vi "Example - Basic IPS-MC.vi"(0 "Mag_Ref":T2, 1 "MB1.T1_Ref":T2, 2 "Temp_present?":bool, 3 "LVL_present?":bool, 4 "Action":T6(ring), 5 "error in (no error)":errorcluster, 6 "LVL_Ref":T2, 7 "ISOBUS address":T5=-1, 8 "Ramp Controls":T9 {"Target Rate (T/min)" format="%_5g"; "Target Field (T)" format="%_5g"; "Target Rate (A/min)" format="%_5g"; "Target Current (A)" format="%_5g"}, 9 "Interval between messages (ms)":i16=100, 10 "Magnet Controls":T10, 11 "Range data":T1, 12 "Display Units":bool caption="AMP/TESLA", 13 "SWITCH\nHEATER":bool) -> (14 "Mag_data":T8 {"Output Voltage (V)" format="%.4f"; "Magnet Current (A)" format="%.4g"; "Output Current (A)" format="%.4g"}, 15 "Environment_data":T7 {"Nitrogen Level (%)" format="%_4f"; "Helium Level (%)" format="%_4f"; "Temperature (K)" format="%_4f"}, 16 "Status":string, 17 "Mode":string, 18 "SW HTR\nCONFIRM":bool, 19 "error out":errorcluster)   [LabVIEW 2013, in "Mercury iXX.lvlib"]
uses:
  Mercury iXX.lvlib
  Public/Libraries/Magnet/Signals/Read/Switch Heater Status (Read).vi
  Public/Libraries/Magnet.lvlib
  Public/Libraries/Magnet/Signals/Read/Current (Read).vi
  Public/Libraries/Magnet/Signals/Read/Persistant Current (Read).vi
  Public/Libraries/Temperature/Signals/Read/Temperature (Read).vi
  Public/Libraries/Temperature.lvlib
  Public/Libraries/Magnet/Configuration/Read/PSU Action Status (Read).vi
  Public/Libraries/Level Meter/Signals/Read/Probe Level Helium (Read).vi
  Public/Libraries/Level Meter.lvlib
  Public/Libraries/Level Meter/Signals/Read/Probe Level Nitrogen (Read).vi
  Public/Libraries/Magnet/Configuration/Read/PSU Status (Read).vi
  Public/Libraries/System/Read/DateTime (Read).vi
  Public/Libraries/System.lvlib
  Public/Libraries/Magnet/Signals/Read/Voltage (Read).vi
  Public/Libraries/Magnet/Controls/PSU Actions.ctl
  Public/Libraries/Magnet/Configuration/Set/PSU Action Status (Set).vi
  Public/Libraries/Magnet/Controls/Switch Heater.ctl
  Public/Libraries/Magnet/Signals/Set/Switch Heater No Check (Set).vi
  Public/Libraries/Magnet/Signals/Set/Target Current (Set).vi
  Public/Libraries/Magnet/Signals/Set/Target Current Rate (Set).vi
  Public/Libraries/Magnet/Signals/Set/Target Field (Set).vi
  Public/Libraries/Magnet/Signals/Set/Target Field Rate (Set).vi
  Public/Controls/Comms Transport Layer.ctl
  Private/Controls/Query Dynamic Reference.ctl
  Public/Controls/Mercury Reference.ctl
  Public/Controls/ISOBus Address.ctl
panel:
  out "Switch TS":timestamp
  out "System Time":string
  in  "Tab Control":enum32{"Link Panel", "Front_Panel", "Error"}(tab)
  out "Voltage (V)":dbl(knob) scale=-10.0..10.0
  out "Current (A)":dbl(knob) scale=-60.0..60.0
  in  "Sw Delay (s)":dbl=30.0 caption="Time Target (s)"
  out "Elapsed\nTime (s)":dbl caption="Elapsed Time (s)"
  out "Magnet Centre Field (T)":dbl format="%.4f"
  out "Output (T) (Field equivalent)":dbl format="%.4f"
  # "Switch Controls"
  # "MercuryiPS-VI"
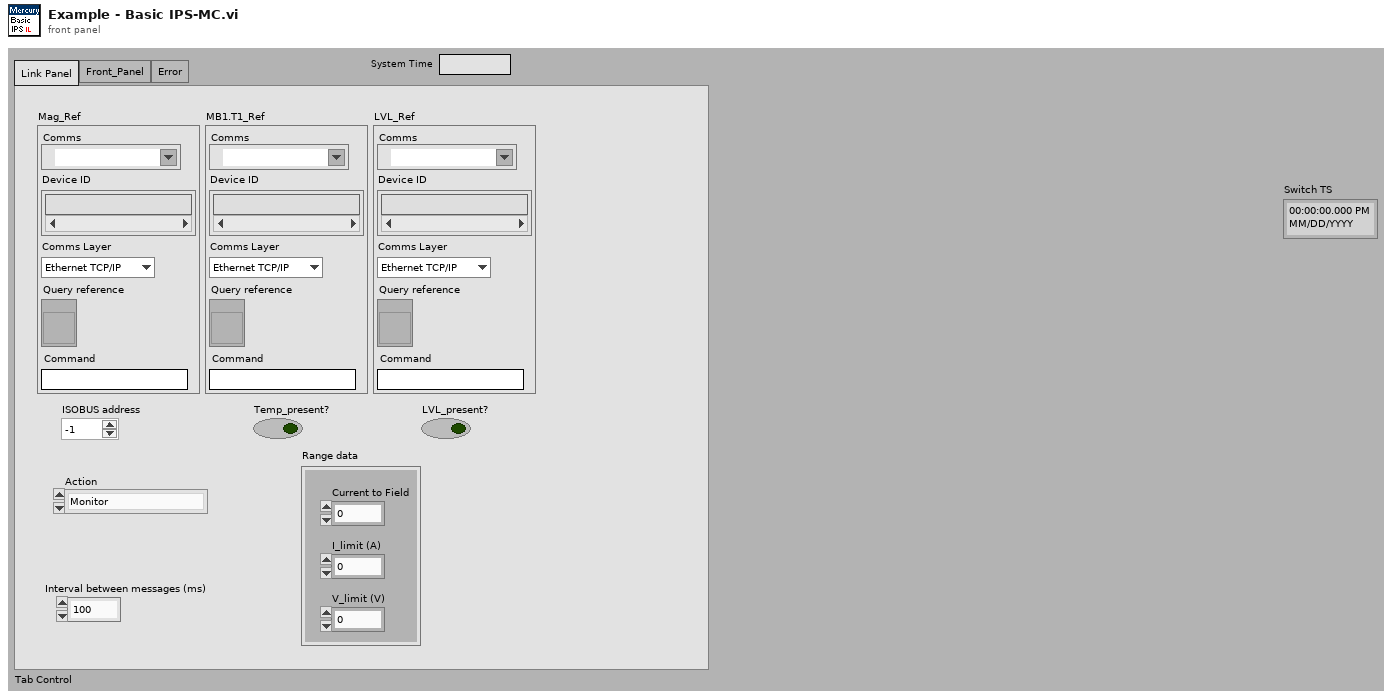
[diagram p1: front panel]
types:
  T1 = cluster{"I_limit (A)":dbl, "V_limit (V)":dbl, "Current to Field":dbl}
  T2 = typedef "Mercury iXX.lvlib/Mercury Reference.ctl" = cluster{"Comms":refnum<visa-resource-name>, "Device ID":string[], "Comms Layer":T3, "Command":string, "Query reference":T4}
  T3 = typedef "Mercury iXX.lvlib/Comms Transport Layer.ctl" = enum16{"Ethernet TCP/IP", "USB", "ISOBus - RS-232", "GPIB"}
  T4 = typedef "Mercury iXX.lvlib/Query Dynamic Reference.ctl" = refnum<vi>
  T5 = typedef "Mercury iXX.lvlib/ISOBus Address.ctl" = i32
  T6 = enum16{"Monitor", "Hold", "Clamp", "To Set", "To Zero", "Switch Heater", "Set Points"}
  T7 = cluster{"Temperature (K)":dbl, "Helium Level (%)":dbl, "Nitrogen Level (%)":dbl}
  T8 = cluster{"Output Current (A)":dbl, "Magnet Current (A)":dbl, "Output Voltage (V)":dbl}
  T9 = cluster{"Target Current (A)":dbl, "Target Rate (A/min)":dbl, "Target Field (T)":dbl, "Target Rate (T/min)":dbl}
  T10 = cluster{"CLAMP":bool, "HOLD":bool, "TO SET":bool, "TO ZERO":bool}
  T11 = typedef "Mercury iXX.lvlib/Magnet.lvlib/PSU Actions.ctl" = string
  T12 = typedef "Mercury iXX.lvlib/Magnet.lvlib/Switch Heater.ctl" = string
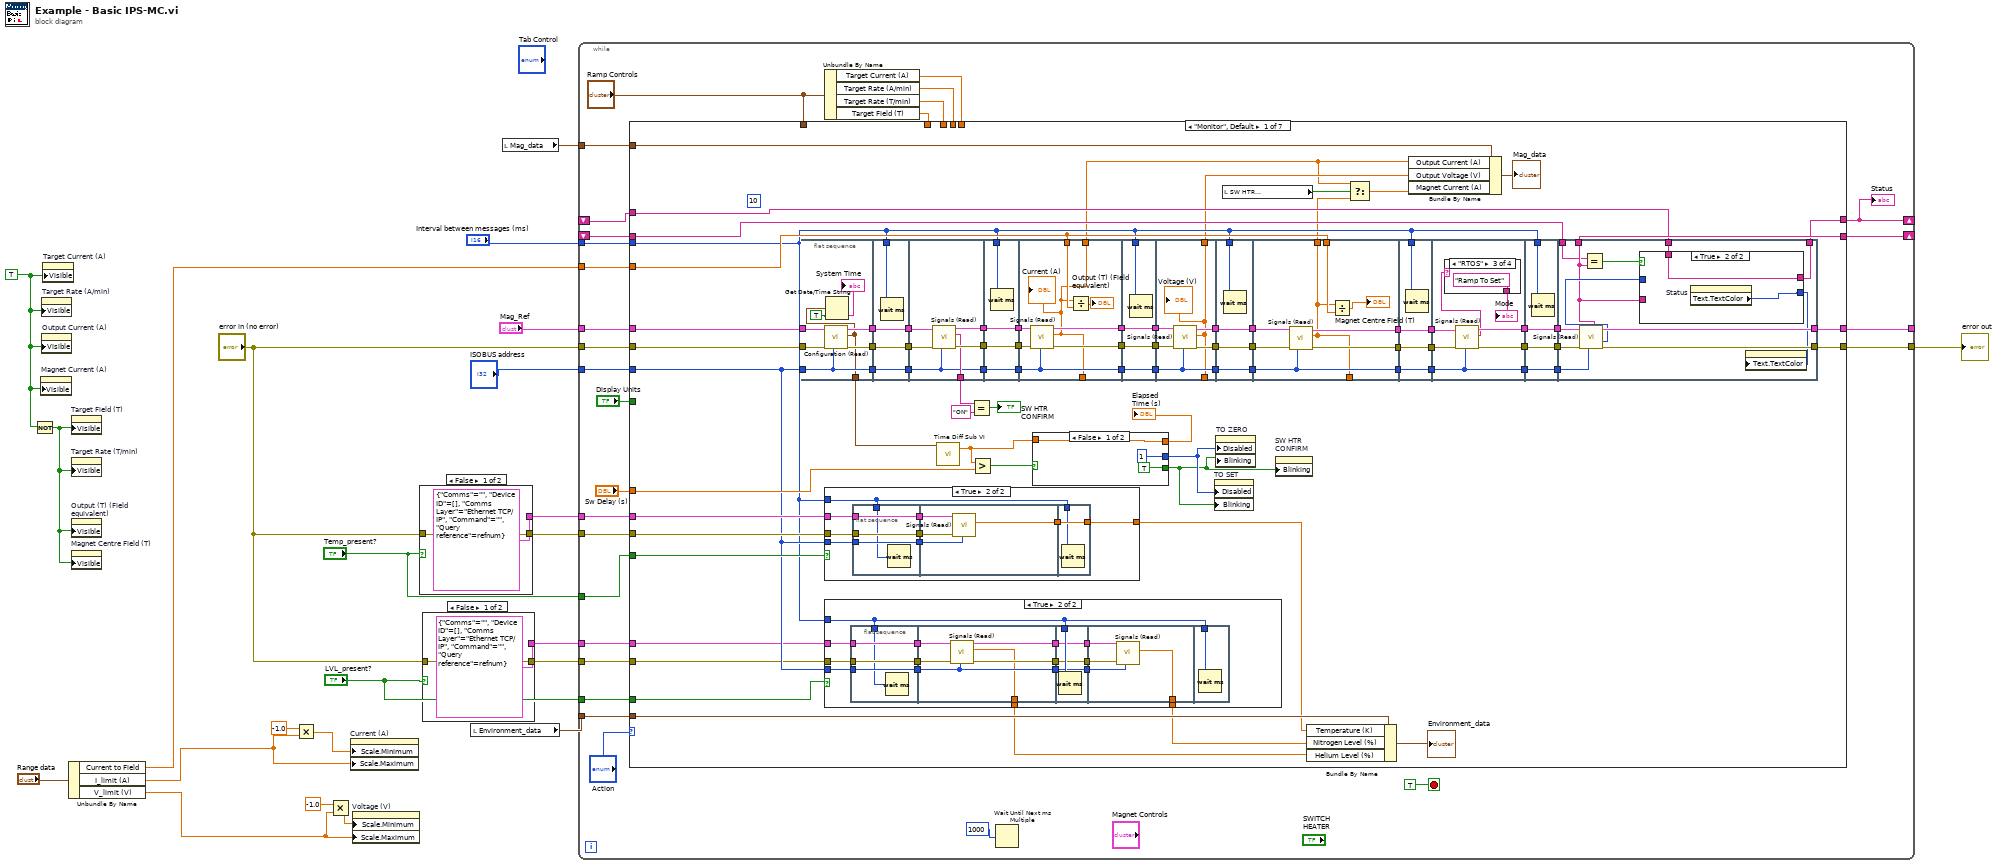
[diagram p0: block diagram]
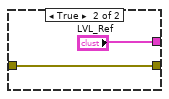
[diagram p2: hidden frame]
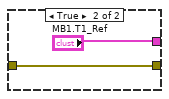
[diagram p3: hidden frame]
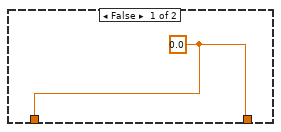
[diagram p4: hidden frame]
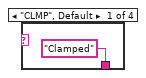
[diagram p5: hidden frame]
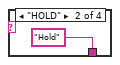
[diagram p6: hidden frame]
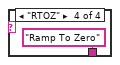
[diagram p7: hidden frame]
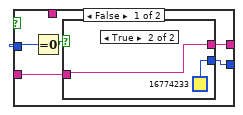
[diagram p8: hidden frame]
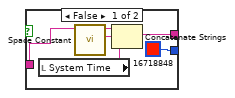
[diagram p9: hidden frame]
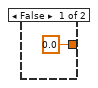
[diagram p10: hidden frame]
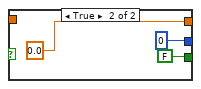
[diagram p11: hidden frame]
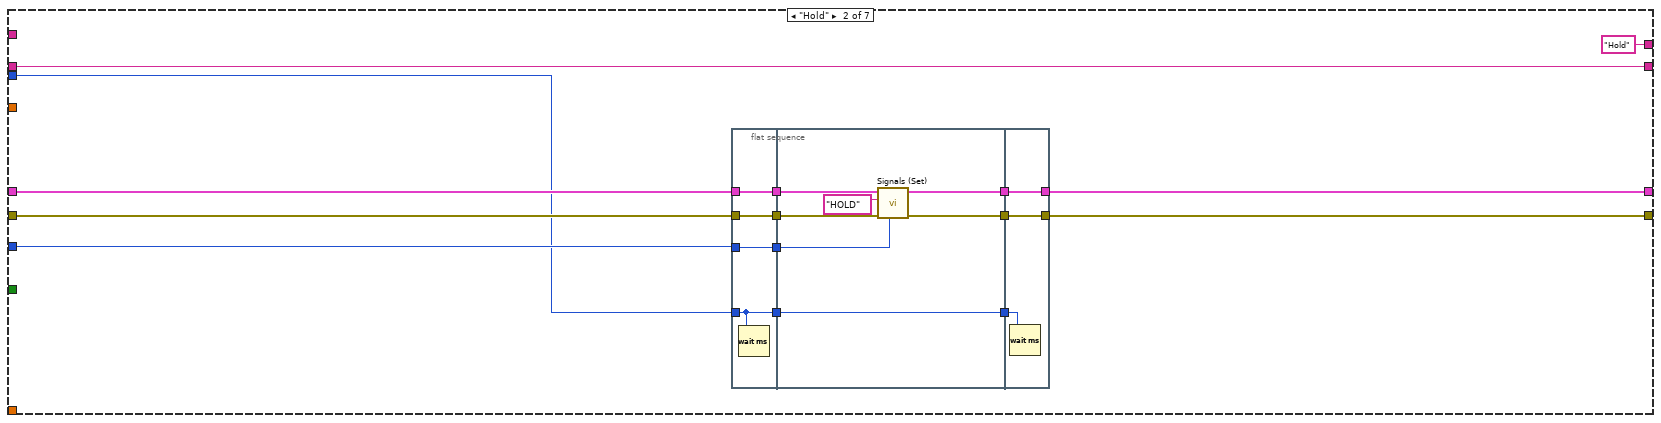
[diagram p12: hidden frame]
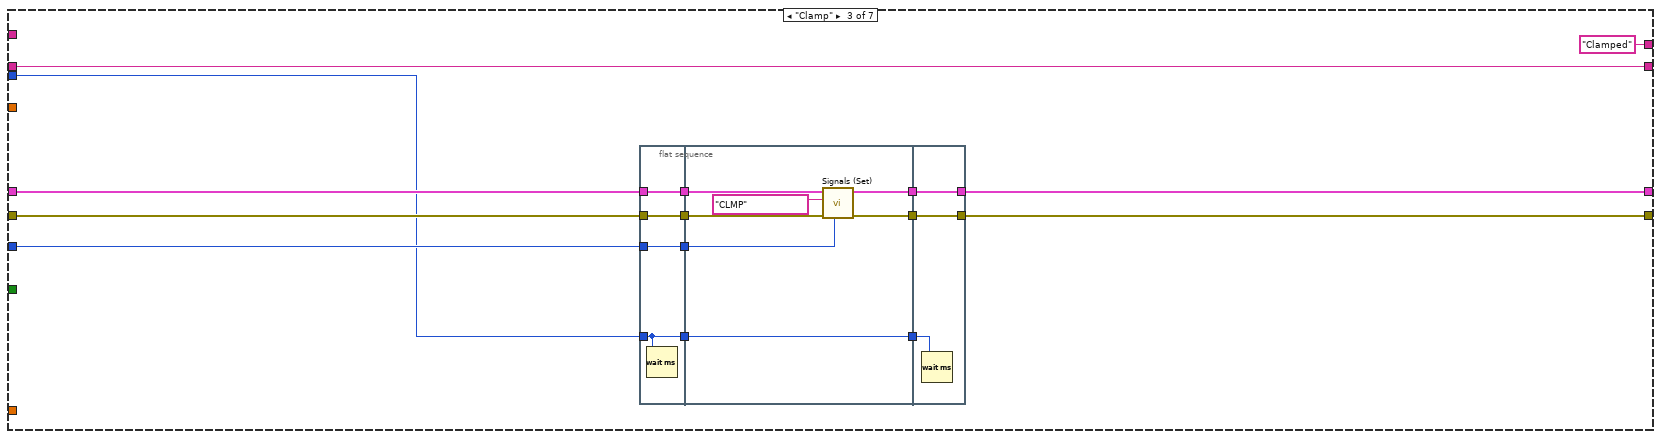
[diagram p13: hidden frame]
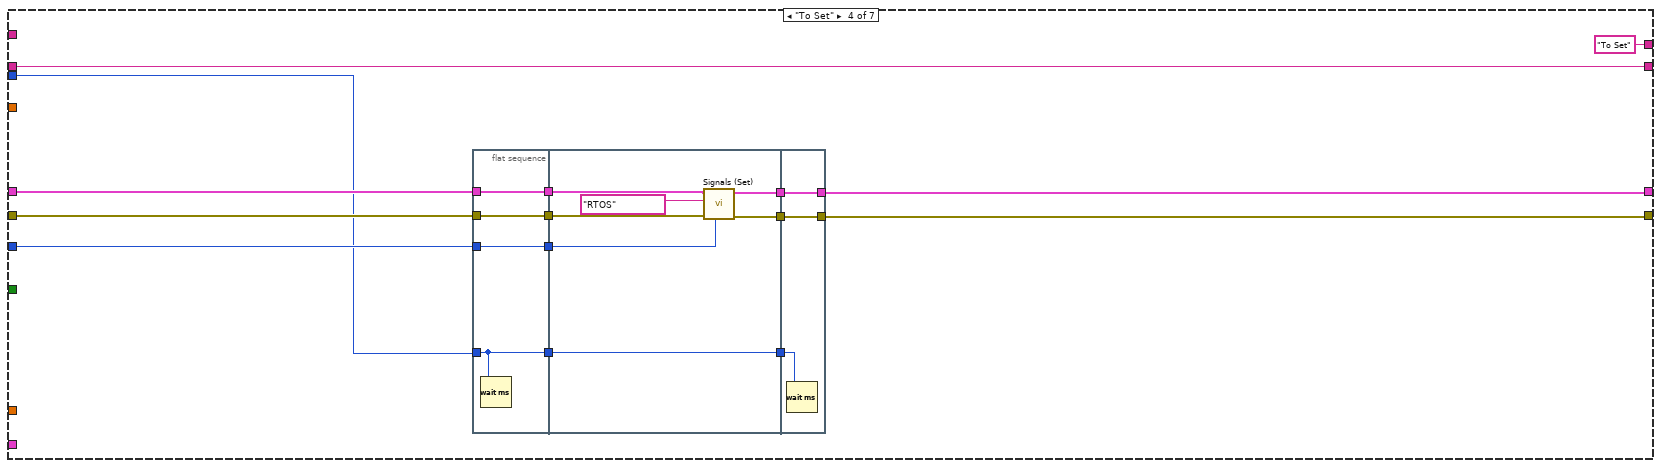
[diagram p14: hidden frame]
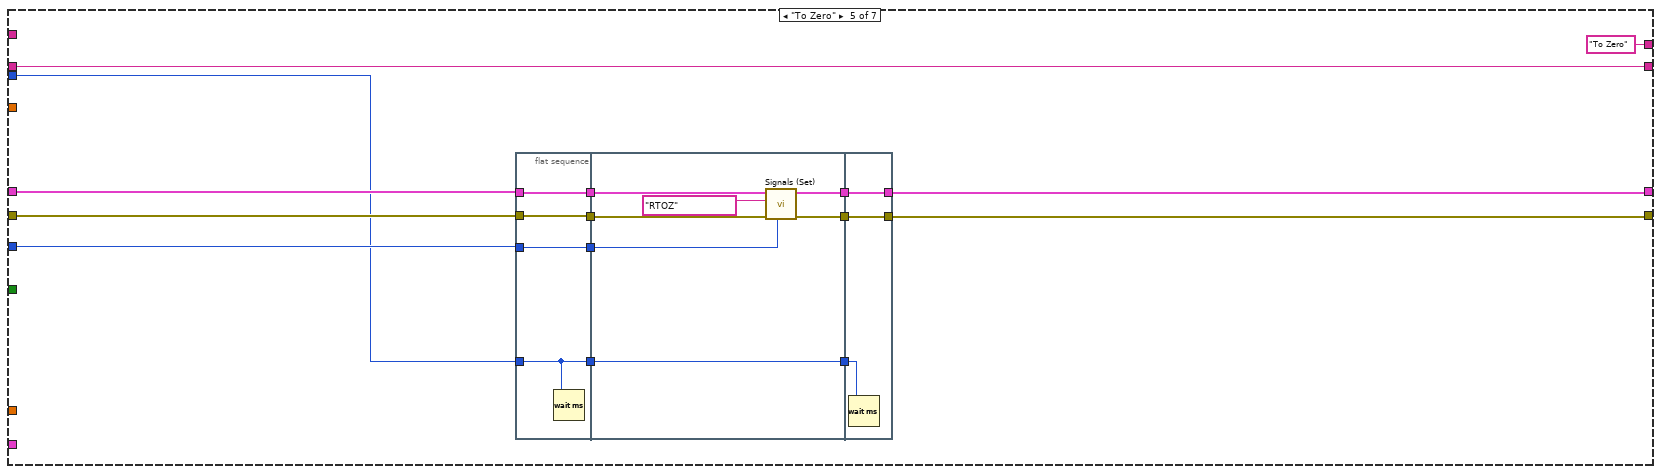
[diagram p15: hidden frame]
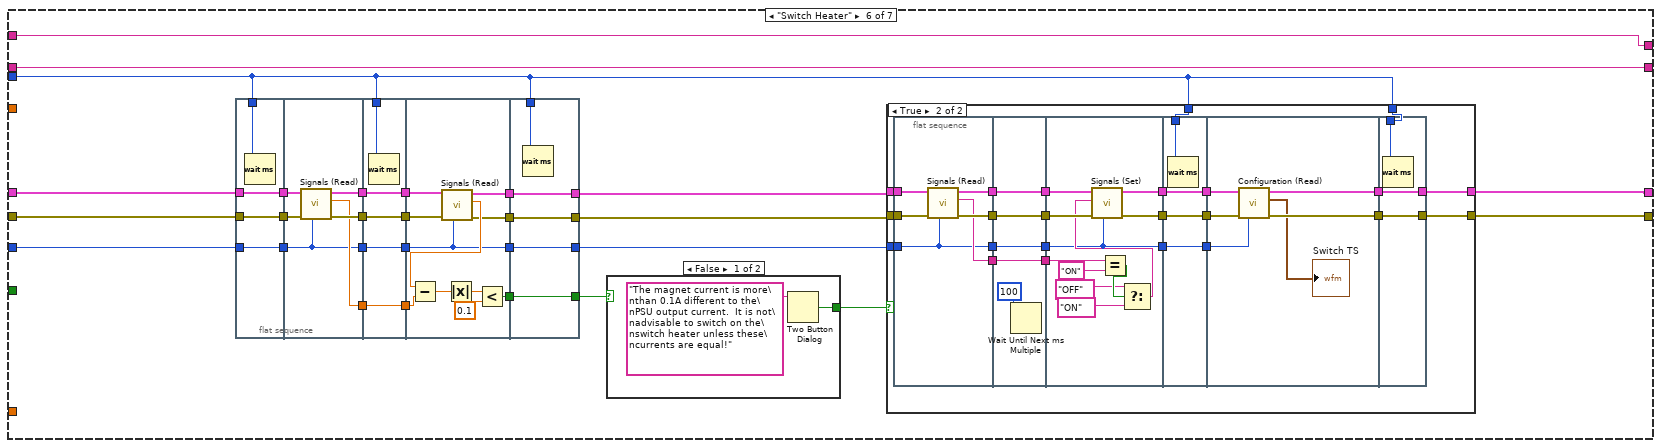
[diagram p16: hidden frame]
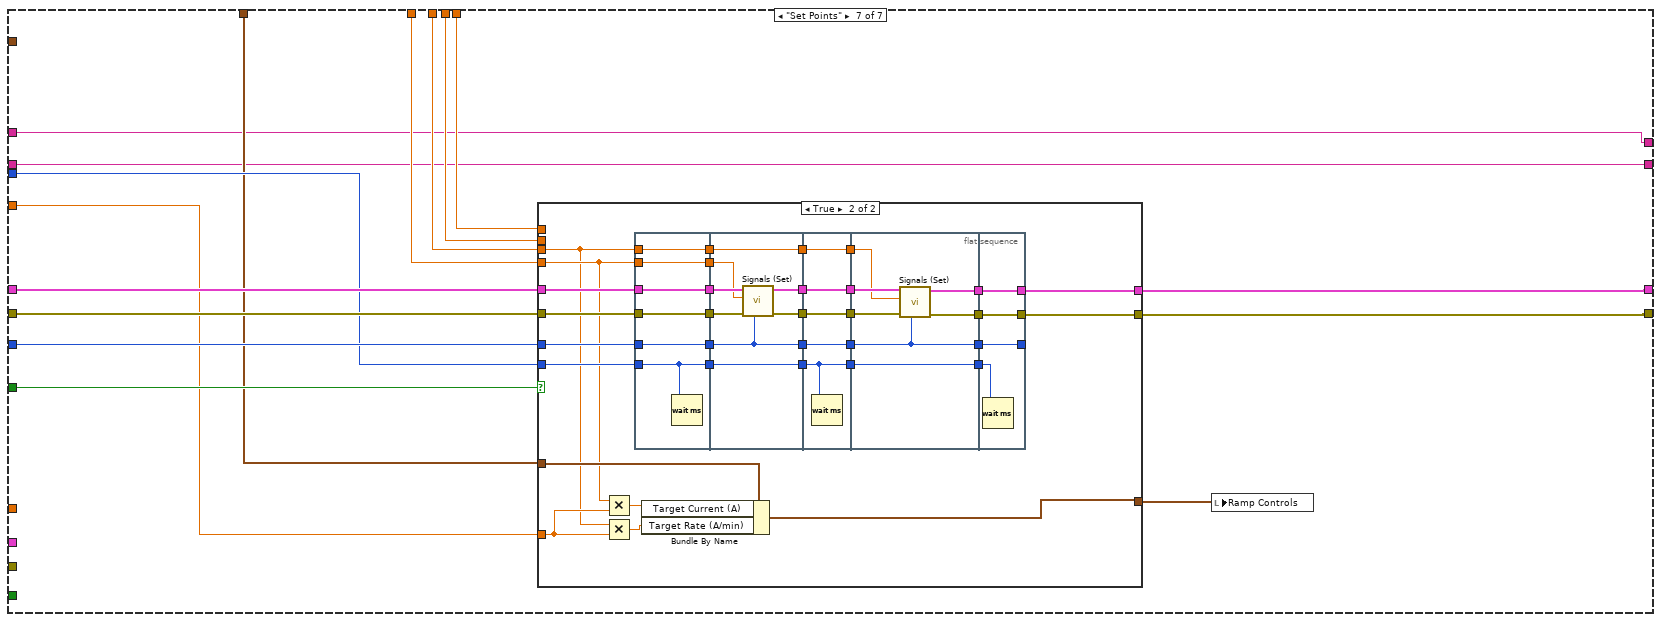
[diagram p19: hidden frame]
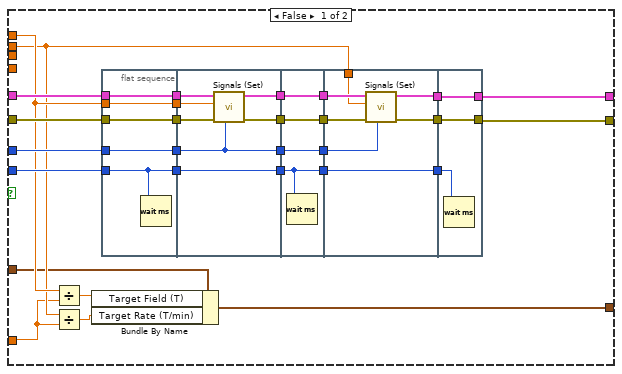
[diagram p20: hidden frame]
diagram:
  w23 = TRUE ("Visible")
  n1 = Not(x=w23) -> (.not. x?=w22:bool)
  n2 = property on="Magnet Current (A)" class="DigNum (strict)"("Visible"=w23) -> ()  [unwired: 2 in, 2 out]
  n3 = property on="Target Rate (A/min)" class="DigNum (strict)"("Visible"=w23) -> ()  [unwired: 2 in, 2 out]
  n4 = property on="Output Current (A)" class="DigNum (strict)"("Visible"=w23) -> ()  [unwired: 2 in, 2 out]
  n5 = property on="Target Current (A)" class="DigNum (strict)"("Visible"=w23) -> ()  [unwired: 2 in, 2 out]
  n6 = Unbundle By Name("Range data") -> ("Current to Field"=w2:dbl, "I_limit (A)"=w4:dbl, "V_limit (V)"=w3:dbl)
  n7 = property on="Target Field (T)" class="DigNum (strict)"("Visible"=w22) -> ()  [unwired: 2 in, 2 out]
  n8 = property on="Target Rate (T/min)" class="DigNum (strict)"("Visible"=w22) -> ()  [unwired: 2 in, 2 out]
  n9 = property on="Output (T) (Field equivalent)" class="DigNum (strict)"("Visible"=w22) -> ()  [unwired: 2 in, 2 out]
  n10 = property on="Magnet Centre Field (T)" class="DigNum (strict)"("Visible"=w22) -> ()  [unwired: 2 in, 2 out]
  n11 = Multiply(x=-1.0, y=w4) -> (x*y=w9:dbl)
  n12 = Multiply(x=-1.0, y=w3) -> (x*y=w10:dbl)
  n13 = property on="Current (A)" class="Knob (strict)"("Scale.Minimum"=w9, "Scale.Maximum"=w4) -> ()  [unwired: 2 in, 2 out]
  n14 = property on="Voltage (V)" class="Knob (strict)"("Scale.Minimum"=w10, "Scale.Maximum"=w3) -> ()  [unwired: 2 in, 2 out]
  n15 = case shown="False" "Temp_present?" {
    tunnel: "error in (no error)" -> [w25 w26]
    tunnel: [T2 {"Comms"="", "Device ID"=[], "Comms Layer"=enum."Ethernet TCP/IP", "Command"="", "Query reference"=refnum} ("MB1.T1_Ref") "MB1.T1_Ref"] -> w14
    tunnel: [w25 w26] -> w20
    frame False {
    }
    frame True {
    }
  }
  n16 = case shown="False" "LVL_present?" {
    tunnel: "error in (no error)" -> [w29 w30]
    tunnel: [T2 {"Comms"="", "Device ID"=[], "Comms Layer"=enum."Ethernet TCP/IP", "Command"="", "Query reference"=refnum} ("LVL_Ref") "LVL_Ref"] -> w19
    tunnel: [w29 w30] -> w18
    frame False {
    }
    frame True {
    }
  }
  n17 = local read "Environment_data"() -> (w16:T7)
  n18 = local read "Mag_data"() -> (w17:T8)
  n19 = while {
    tunnel: "Mag_Ref" -> [w59]
    tunnel: "error in (no error)" -> [w58]
    tunnel: [w57] -> _
    tunnel: [w56] -> w1
    tunnel: w2 -> [w54]
    tunnel: w14 -> [w47]
    tunnel: w20 -> [w46]
    tunnel: "Temp_present?" -> [w48]
    tunnel: "ISOBUS address" -> [w45]
    tunnel: "Interval between messages (ms)" -> [w44]
    tunnel: w19 -> [w43]
    tunnel: w18 -> [w42]
    tunnel: "LVL_present?" -> [w41]
    shift-right: [w40] -> _
    shift-left: _ -> [w39]
    shift-right: [w35] -> _
    shift-left: _ -> [w38]
    tunnel: w17 -> [w33]
    tunnel: w16 -> [w32]
    stop <- TRUE stop-if-true
    n20 = Unbundle By Name("Ramp Controls") -> ("Target Current (A)"=w51:dbl, "Target Rate (A/min)"=w52:dbl, "Target Rate (T/min)"=w50:dbl, "Target Field (T)"=w49:dbl)
    n21 = case shown="\"Monitor\", Default" "Action" {
      tunnel: w59 -> [w135 w301 w330 w359 w388 w422 w547]
      tunnel: w58 -> [w134 w300 w329 w358 w387 w421 w546]
      tunnel: [w133 w297 w326 w355 w384 w413 w535] -> w57
      tunnel: [w132 w296 w325 w354 w383 w412 w534] -> w56
      tunnel: "Sw Delay (s)" -> [w131 _ _ _ _ _ _]
      tunnel: w54 -> [w130 _ _ _ _ _ w537]
      tunnel: "Display Units" -> [_ _ _ _ _ _ w539]
      tunnel: w52 -> [_ _ _ _ _ _ w544]
      tunnel: w51 -> [_ _ _ _ _ _ w545]
      tunnel: w50 -> [_ _ _ _ _ _ w543]
      tunnel: w49 -> [_ _ _ _ _ _ w542]
      tunnel: w48 -> [w129 _ _ _ _ _ _]
      tunnel: w47 -> [w128 _ _ _ _ _ _]
      tunnel: w46 -> [w127 _ _ _ _ _ _]
      tunnel: w45 -> [w126 w299 w328 w357 w386 w420 w541]
      tunnel: w44 -> [w125 w298 w327 w356 w385 w414 w540]
      tunnel: w43 -> [w124 _ _ _ _ _ _]
      tunnel: w42 -> [w123 _ _ _ _ _ _]
      tunnel: w41 -> [w122 _ _ _ _ _ _]
      tunnel: [w121 w295 w324 w353 w382 w411 w533] -> w40
      tunnel: w39 -> [w120 w295 w324 w353 w382 w411 w533]
      tunnel: [w119 "Hold" ("Status") "Clamped" ("Status") "To Set" ("Status") "To Zero" ("Status") w410 w532] -> w35
      tunnel: w38 -> [w118 _ _ _ _ w410 w532]
      tunnel: "Ramp Controls" -> [_ _ _ _ _ _ w538]
      tunnel: w33 -> [w72 _ _ _ _ _ _]
      tunnel: w32 -> [w69 _ _ _ _ _ _]
      frame "Monitor", Default {
        (unwired) 10
        n22 = flat-sequence {
          tunnel: [w173] -> w74
          tunnel: w135 -> [w178]
          tunnel: w134 -> [w177]
          tunnel: [w176] -> w117
          tunnel: [w175] -> w116
          tunnel: w126 -> [w174]
          tunnel: [w174] -> w115
          tunnel: w117 -> [w182]
          tunnel: w116 -> [w181]
          tunnel: [w182] -> w114
          tunnel: [w181] -> w113
          tunnel: [w180] -> w112
          tunnel: w115 -> [w180]
          tunnel: w125 -> [w179]
          tunnel: w114 -> [w187]
          tunnel: w113 -> [w188]
          tunnel: [w184] -> w75
          tunnel: [w186] -> w111
          tunnel: [w185] -> w110
          tunnel: w112 -> [w183]
          tunnel: [w183] -> w109
          tunnel: w111 -> [w192]
          tunnel: w110 -> [w191]
          tunnel: [w192] -> w108
          tunnel: [w191] -> w107
          tunnel: [w190] -> w106
          tunnel: w109 -> [w190]
          tunnel: w125 -> [w189]
          tunnel: w108 -> [w200]
          tunnel: w107 -> [w199]
          tunnel: w130 -> [w197]
          tunnel: [w196] -> w105
          tunnel: [w195] -> w104
          tunnel: [w193] -> _
          tunnel: w106 -> [w194]
          tunnel: [w194] -> w103
          tunnel: [w193] -> w62
          tunnel: w105 -> [w204]
          tunnel: w104 -> [w203]
          tunnel: [w204] -> w102
          tunnel: [w203] -> w101
          tunnel: [w202] -> w100
          tunnel: w103 -> [w202]
          tunnel: w125 -> [w201]
          tunnel: w102 -> [w210]
          tunnel: w101 -> [w209]
          tunnel: [w205] -> _
          tunnel: [w208] -> w99
          tunnel: [w207] -> w98
          tunnel: w100 -> [w206]
          tunnel: [w206] -> w97
          tunnel: [w205] -> w70
          tunnel: w99 -> [w214]
          tunnel: w98 -> [w213]
          tunnel: [w214] -> w96
          tunnel: [w213] -> w95
          tunnel: [w212] -> w94
          tunnel: w97 -> [w212]
          tunnel: w125 -> [w211]
          tunnel: w96 -> [w222]
          tunnel: w95 -> [w221]
          tunnel: w130 -> [w217]
          tunnel: [w215] -> _
          tunnel: [w220] -> w93
          tunnel: [w219] -> w92
          tunnel: w94 -> [w216]
          tunnel: [w216] -> w91
          tunnel: [w215] -> w64
          tunnel: w93 -> [w226]
          tunnel: w92 -> [w225]
          tunnel: [w226] -> w90
          tunnel: [w225] -> w89
          tunnel: [w224] -> w88
          tunnel: w91 -> [w224]
          tunnel: w125 -> [w223]
          tunnel: w90 -> [w232]
          tunnel: w89 -> [w233]
          tunnel: w88 -> [w229]
          tunnel: [w231] -> w87
          tunnel: [w230] -> w86
          tunnel: [w229] -> w85
          tunnel: w87 -> [w241]
          tunnel: w86 -> [w240]
          tunnel: w125 -> [w239]
          tunnel: [w241] -> w84
          tunnel: [w240] -> w83
          tunnel: [w238] -> w82
          tunnel: w85 -> [w238]
          tunnel: [w250] -> w132
          tunnel: [w251] -> w133
          tunnel: w84 -> [w252]
          tunnel: w83 -> [w253]
          tunnel: w82 -> [w249]
          tunnel: [w245] -> w121
          tunnel: w120 -> [w244]
          tunnel: [w243] -> w119
          tunnel: w118 -> [w242]
          frame #0 {
            n23 = call-poly "Configuration (Read).vi"("ISOBUS address"=w174, "error in"=w177, "Mercury Reference In"=w178) -> ("error out"=w175:errorcluster, "time stamp"=w173:timestamp, "Mercury Reference Out"=w176:T2)  [unwired: 6 out]
            n24 = Get Date/Time String(seconds (now)=w173, want seconds? (F)=TRUE) -> (time string=→"System Time":string)  [unwired: 1 in, 1 out]
          }
          frame #1 {
            n25 = Wait (ms)(milliseconds to wait=w179) -> ()  [unwired: 1 out]
          }
          frame #2 {
            n26 = call-poly "Signals (Read).vi"("ISOBUS address"=w183, "error in"=w188, "Mercury Reference In"=w187) -> ("error out"=w185:errorcluster, "Switch Heater Status"=w184:string, "Mercury Reference Out"=w186:T2)  [unwired: 6 out]
          }
          frame #3 {
            n27 = Wait (ms)(milliseconds to wait=w189) -> ()  [unwired: 1 out]
          }
          frame #4 {
            n28 = call-poly "Signals (Read).vi"("ISOBUS address"=w194, "error in"=w199, "Mercury Reference In"=w200) -> ("error out"=w195:errorcluster, "Current"=w193:dbl, "Mercury Reference Out"=w196:T2)  [unwired: 6 out]
            "Current (A)" <- w193
            n29 = Divide(x=w193, y=w197) -> (x/y=→"Output (T) (Field equivalent)":dbl)
          }
          frame #5 {
            n30 = Wait (ms)(milliseconds to wait=w201) -> ()  [unwired: 1 out]
          }
          frame #6 {
            n31 = call-poly "Signals (Read).vi"("ISOBUS address"=w206, "error in"=w209, "Mercury Reference In"=w210) -> ("error out"=w207:errorcluster, "Voltage"=w205:dbl, "Mercury Reference Out"=w208:T2)  [unwired: 6 out]
            "Voltage (V)" <- w205
          }
          frame #7 {
            n32 = Wait (ms)(milliseconds to wait=w211) -> ()  [unwired: 1 out]
          }
          frame #8 {
            n33 = call-poly "Signals (Read).vi"("ISOBUS address"=w216, "error in"=w221, "Mercury Reference In"=w222) -> ("error out"=w220:errorcluster, "Persistant Current"=w215:dbl, "Mercury Reference Out"=w219:T2)  [unwired: 6 out]
            n34 = Divide(x=w215, y=w217) -> (x/y=→"Magnet Centre Field (T)":dbl)
          }
          frame #9 {
            n35 = Wait (ms)(milliseconds to wait=w223) -> ()  [unwired: 1 out]
          }
          frame #10 {
            n36 = call-poly "Signals (Read).vi"("ISOBUS address"=w229, "error in"=w232, "Mercury Reference In"=w233) -> ("error out"=w230:errorcluster, "PSU Act Stat"=w228:T11, "Mercury Reference Out"=w231:T2)  [unwired: 6 out]
            n37 = case shown="\"RTOS\"" w228 {
              tunnel: ["Clamped" "Hold" "Ramp To Set" "Ramp To Zero"] -> w227
              frame "CLMP", Default {
              }
              frame "HOLD" {
              }
              frame "RTOS" {
              }
              frame "RTOZ" {
              }
            }
            "Mode" <- w227
          }
          frame #11 {
            n38 = Wait (ms)(milliseconds to wait=w239) -> ()  [unwired: 1 out]
          }
          frame #12 {
            n39 = call-poly "Signals (Read).vi"("ISOBUS address"=w249, "error in"=w253, "Mercury Reference In"=w252) -> ("error out"=w250:errorcluster, "Status Hex value"=w248:i32, "Mercury Reference Out"=w251:T2, "Status"=w245:string)  [unwired: 3 in, 2 out]
            n40 = Equal?(x=w244, y=w245) -> (x = y?=w246:bool)
            n41 = case shown="True" w246 {
              tunnel: w248 -> [w258 _]
              tunnel: w245 -> [w257 _]
              tunnel: [w255 w267] -> w243
              tunnel: [w254 w266] -> w247
              tunnel: w242 -> [_ w267]
              frame False {
                n42 = Equal To 0?(x=w258) -> (x = 0?=w256:bool)
                n43 = case shown="True" w256 {
                  tunnel: w257 -> [w260 w264]
                  tunnel: [w259 w264] -> w255
                  tunnel: [u32 16718848 ("Text.Text Colors:Text Color") u32 16774233 ("Text.Text Colors:Text Color")] -> w254
                  frame False {
                    n44 = local read "System Time"() -> (w262:string)
                    n45 = call <vilib>:"Space Constant.vi"() -> ("String"=w261:string)
                    n46 = Concatenate Strings(w260, w261, w262) -> (w259:string)
                  }
                  frame True {
                  }
                }
              }
              frame True {
                n47 = property on="Status" class="Str"() -> ("Text.TextColor"=w266:u32)  [unwired: 2 in, 2 out]
              }
            }
            n48 = property on="Status" class="Str"("Text.TextColor"=w247) -> ()  [unwired: 2 in, 2 out]
          }
        }
        n49 = case shown="True" w129 {
          tunnel: w128 -> [_ w277]
          tunnel: w127 -> [_ w276]
          tunnel: [0.0 ("Temperature") w275] -> w65
          tunnel: w126 -> [_ w274]
          tunnel: w125 -> [_ w269]
          frame False {
          }
          frame True {
            n50 = flat-sequence {
              tunnel: w274 -> [w279]
              tunnel: w276 -> [w280]
              tunnel: w277 -> [w281]
              tunnel: [w281] -> w272
              tunnel: [w280] -> w271
              tunnel: [w279] -> w270
              tunnel: w269 -> [w278]
              tunnel: [w283] -> w273
              tunnel: w272 -> [w285]
              tunnel: w271 -> [w284]
              tunnel: w270 -> [w282]
              tunnel: [w287] -> w275
              tunnel: w273 -> [w287]
              tunnel: w269 -> [w286]
              frame #0 {
                n51 = Wait (ms)(milliseconds to wait=w278) -> ()  [unwired: 1 out]
              }
              frame #1 {
                n52 = call-poly "Signals (Read).vi"("ISOBUS address"=w282, "error in"=w284, "Mercury Reference In"=w285) -> ("Temperature"=w283:dbl)  [unwired: 4 in, 4 out]
              }
              frame #2 {
                n53 = Wait (ms)(milliseconds to wait=w286) -> ()  [unwired: 1 out]
              }
            }
          }
        }
        n54 = case shown="True" w122 {
          tunnel: w124 -> [_ w151]
          tunnel: w123 -> [_ w150]
          tunnel: w126 -> [_ w149]
          tunnel: w125 -> [_ w139]
          tunnel: [w136 w138] -> w67
          tunnel: [w136 w137] -> w66
          frame False {
            w136 = 0.0 ("Temperature")
          }
          frame True {
            n55 = flat-sequence {
              tunnel: w149 -> [w153]
              tunnel: w150 -> [w154]
              tunnel: w151 -> [w155]
              tunnel: [w155] -> w148
              tunnel: [w154] -> w147
              tunnel: [w153] -> w146
              tunnel: w139 -> [w152]
              tunnel: w148 -> [w161]
              tunnel: w147 -> [w160]
              tunnel: w146 -> [w157]
              tunnel: [w159] -> w144
              tunnel: [w158] -> w142
              tunnel: [w157] -> w140
              tunnel: [w156] -> w137
              tunnel: w139 -> [w165]
              tunnel: [w164] -> w145
              tunnel: w144 -> [w164]
              tunnel: [w163] -> w143
              tunnel: w142 -> [w163]
              tunnel: [w162] -> w141
              tunnel: w140 -> [w162]
              tunnel: w145 -> [w169]
              tunnel: w143 -> [w168]
              tunnel: w141 -> [w167]
              tunnel: [w166] -> w138
              tunnel: w139 -> [w170]
              frame #0 {
                n56 = Wait (ms)(milliseconds to wait=w152) -> ()  [unwired: 1 out]
              }
              frame #1 {
                n57 = call-poly "Signals (Read).vi"("ISOBUS address"=w157, "error in"=w160, "Mercury Reference In"=w161) -> ("error out"=w158:errorcluster, "Level"=w156:dbl, "Mercury Reference Out"=w159:T2)  [unwired: 4 in, 2 out]
              }
              frame #2 {
                n58 = Wait (ms)(milliseconds to wait=w165) -> ()  [unwired: 1 out]
              }
              frame #3 {
                n59 = call-poly "Signals (Read).vi"("ISOBUS address"=w167, "error in"=w168, "Mercury Reference In"=w169) -> ("Level"=w166:dbl)  [unwired: 4 in, 4 out]
              }
              frame #4 {
                n60 = Wait (ms)(milliseconds to wait=w170) -> ()  [unwired: 1 out]
              }
            }
          }
        }
        n61 = call "Time Diff Sub VI.vi"("Current Time Stamp"=w74) -> ("Time Diff"=w73:dbl)  [unwired: 3 in, 1 out]
        n62 = Equal?(x=w75, y="ON") -> (x = y?=→"SW HTR\nCONFIRM":bool)
        n63 = Greater?(x=w73, y=w131) -> (0:w79:bool)
        n64 = case shown="False" w79 {
          tunnel: [w290 0.0 ("Elapsed\nTime (s)")] -> w78
          tunnel: w73 -> [w290 _]
          tunnel: [TRUE ("Blinking") FALSE ("Blinking")] -> w76
          tunnel: [u8 1 ("Disabled") u8 0 ("Disabled")] -> w77
          frame False {
          }
          frame True {
          }
        }
        "Elapsed\nTime (s)" <- w78
        n65 = property on="TO SET" class="Bool"("Disabled"=w77, "Blinking"=w76) -> ()  [unwired: 2 in, 2 out]
        n66 = property on="TO ZERO" class="Bool"("Disabled"=w77, "Blinking"=w76) -> ()  [unwired: 2 in, 2 out]
        n67 = local read "SW HTR\nCONFIRM"() -> (w61:bool)
        n68 = property on="SW HTR\nCONFIRM" class="Bool (strict)"("Blinking"=w76) -> ()  [unwired: 2 in, 2 out]
        n69 = Bundle By Name(cluster=w69, "Temperature (K)"=w65, "Nitrogen Level (%)"=w67, "Helium Level (%)"=w66) -> (→"Environment_data":T7)
        n70 = Select(t=w62, s=w61, f=w64) -> (s? t:f=w63:dbl)
        n71 = Bundle By Name(cluster=w72, "Output Current (A)"=w62, "Output Voltage (V)"=w70, "Magnet Current (A)"=w63) -> (→"Mag_data":T8)
      }
      frame "Hold" {
        n72 = flat-sequence {
          tunnel: w299 -> [w310]
          tunnel: w301 -> [w311]
          tunnel: w300 -> [w312]
          tunnel: [w312] -> w308
          tunnel: [w311] -> w307
          tunnel: [w310] -> w306
          tunnel: [w309] -> w305
          tunnel: w298 -> [w309]
          tunnel: w308 -> [w319]
          tunnel: w307 -> [w318]
          tunnel: w306 -> [w314]
          tunnel: [w317] -> w304
          tunnel: [w316] -> w303
          tunnel: [w313] -> w302
          tunnel: w305 -> [w313]
          tunnel: [w321] -> w296
          tunnel: [w322] -> w297
          tunnel: w304 -> [w322]
          tunnel: w303 -> [w321]
          tunnel: w302 -> [w320]
          frame #0 {
            n73 = Wait (ms)(milliseconds to wait=w309) -> ()  [unwired: 1 out]
          }
          frame #1 {
            n74 = call-poly "Signals (Set).vi"("ISOBUS address"=w314, "error in"=w319, "PSU Act Stat"=T11 "HOLD", "Mercury Reference In"=w318) -> ("error out"=w316:errorcluster, "Mercury Reference Out"=w317:T2)  [unwired: 6 out]
          }
          frame #2 {
            n75 = Wait (ms)(milliseconds to wait=w320) -> ()  [unwired: 1 out]
          }
        }
      }
      frame "Clamp" {
        n76 = flat-sequence {
          tunnel: w328 -> [w339]
          tunnel: w329 -> [w340]
          tunnel: w330 -> [w341]
          tunnel: [w341] -> w337
          tunnel: [w340] -> w336
          tunnel: [w339] -> w335
          tunnel: [w338] -> w334
          tunnel: w327 -> [w338]
          tunnel: w337 -> [w348]
          tunnel: w336 -> [w347]
          tunnel: w335 -> [w343]
          tunnel: [w346] -> w333
          tunnel: [w345] -> w332
          tunnel: [w342] -> w331
          tunnel: w334 -> [w342]
          tunnel: [w350] -> w325
          tunnel: [w351] -> w326
          tunnel: w333 -> [w351]
          tunnel: w332 -> [w350]
          tunnel: w331 -> [w349]
          frame #0 {
            n77 = Wait (ms)(milliseconds to wait=w338) -> ()  [unwired: 1 out]
          }
          frame #1 {
            n78 = call-poly "Signals (Set).vi"("ISOBUS address"=w343, "error in"=w347, "PSU Act Stat"=T11 "CLMP", "Mercury Reference In"=w348) -> ("error out"=w345:errorcluster, "Mercury Reference Out"=w346:T2)  [unwired: 6 out]
          }
          frame #2 {
            n79 = Wait (ms)(milliseconds to wait=w349) -> ()  [unwired: 1 out]
          }
        }
      }
      frame "To Set" {
        n80 = flat-sequence {
          tunnel: w357 -> [w368]
          tunnel: w358 -> [w369]
          tunnel: w359 -> [w370]
          tunnel: [w370] -> w366
          tunnel: [w369] -> w365
          tunnel: [w368] -> w364
          tunnel: [w367] -> w363
          tunnel: w356 -> [w367]
          tunnel: w366 -> [w377]
          tunnel: w365 -> [w376]
          tunnel: w364 -> [w372]
          tunnel: [w375] -> w362
          tunnel: [w374] -> w361
          tunnel: [w371] -> w360
          tunnel: w363 -> [w371]
          tunnel: [w379] -> w354
          tunnel: [w380] -> w355
          tunnel: w362 -> [w380]
          tunnel: w361 -> [w379]
          tunnel: w360 -> [w378]
          frame #0 {
            n81 = Wait (ms)(milliseconds to wait=w367) -> ()  [unwired: 1 out]
          }
          frame #1 {
            n82 = call-poly "Signals (Set).vi"("ISOBUS address"=w372, "error in"=w376, "PSU Act Stat"=T11 "RTOS", "Mercury Reference In"=w377) -> ("error out"=w374:errorcluster, "Mercury Reference Out"=w375:T2)  [unwired: 6 out]
          }
          frame #2 {
            n83 = Wait (ms)(milliseconds to wait=w378) -> ()  [unwired: 1 out]
          }
        }
      }
      frame "To Zero" {
        n84 = flat-sequence {
          tunnel: w386 -> [w398]
          tunnel: w388 -> [w399]
          tunnel: [w399] -> w395
          tunnel: [w396] -> w394
          tunnel: [w398] -> w393
          tunnel: [w397] -> w392
          tunnel: w385 -> [w397]
          tunnel: w387 -> [w396]
          tunnel: w395 -> [w406]
          tunnel: w394 -> [w405]
          tunnel: w393 -> [w401]
          tunnel: [w404] -> w391
          tunnel: [w403] -> w390
          tunnel: [w400] -> w389
          tunnel: w392 -> [w400]
          tunnel: [w408] -> w383
          tunnel: [w409] -> w384
          tunnel: w391 -> [w409]
          tunnel: w390 -> [w408]
          tunnel: w389 -> [w407]
          frame #0 {
            n85 = Wait (ms)(milliseconds to wait=w397) -> ()  [unwired: 1 out]
          }
          frame #1 {
            n86 = call-poly "Signals (Set).vi"("ISOBUS address"=w401, "error in"=w405, "PSU Act Stat"=T11 "RTOZ", "Mercury Reference In"=w406) -> ("error out"=w403:errorcluster, "Mercury Reference Out"=w404:T2)  [unwired: 6 out]
          }
          frame #2 {
            n87 = Wait (ms)(milliseconds to wait=w407) -> ()  [unwired: 1 out]
          }
        }
      }
      frame "Switch Heater" {
        n88 = flat-sequence {
          tunnel: w420 -> [w502]
          tunnel: w421 -> [w503]
          tunnel: w422 -> [w504]
          tunnel: [w504] -> w437
          tunnel: [w503] -> w436
          tunnel: [w502] -> w435
          tunnel: w414 -> [w501]
          tunnel: [w510] -> w434
          tunnel: [w509] -> w433
          tunnel: [w506] -> w432
          tunnel: [w505] -> w431
          tunnel: w437 -> [w508]
          tunnel: w436 -> [w507]
          tunnel: w435 -> [w505]
          tunnel: w434 -> [w515]
          tunnel: w433 -> [w514]
          tunnel: w432 -> [w513]
          tunnel: [w515] -> w430
          tunnel: [w514] -> w429
          tunnel: [w513] -> w428
          tunnel: [w512] -> w427
          tunnel: w431 -> [w512]
          tunnel: w414 -> [w511]
          tunnel: w430 -> [w520]
          tunnel: w429 -> [w519]
          tunnel: w428 -> [w526]
          tunnel: w427 -> [w516]
          tunnel: [w521] -> w426
          tunnel: [w518] -> w425
          tunnel: [w517] -> w424
          tunnel: [w516] -> w423
          tunnel: [w528] -> w416
          tunnel: [w529] -> w417
          tunnel: [w530] -> w418
          tunnel: [w531] -> w419
          tunnel: w426 -> [w531]
          tunnel: w425 -> [w530]
          tunnel: w424 -> [w529]
          tunnel: w423 -> [w528]
          tunnel: w414 -> [w527]
          frame #0 {
            n89 = Wait (ms)(milliseconds to wait=w501) -> ()  [unwired: 1 out]
          }
          frame #1 {
            n90 = call-poly "Signals (Read).vi"("ISOBUS address"=w505, "error in"=w507, "Mercury Reference In"=w508) -> ("error out"=w509:errorcluster, "Current"=w506:dbl, "Mercury Reference Out"=w510:T2)  [unwired: 6 out]
          }
          frame #2 {
            n91 = Wait (ms)(milliseconds to wait=w511) -> ()  [unwired: 1 out]
          }
          frame #3 {
            n92 = call-poly "Signals (Read).vi"("ISOBUS address"=w516, "error in"=w519, "Mercury Reference In"=w520) -> ("error out"=w517:errorcluster, "Persistant Current"=w525:dbl, "Mercury Reference Out"=w518:T2)  [unwired: 6 out]
            n93 = Subtract(x=w525, y=w526) -> (x-y=w524:dbl)
            n94 = Absolute Value(x=w524) -> (abs(x)=w523:dbl)
            n95 = Less?(x=w523, y=0.1) -> (x < y?=w521:bool)
          }
          frame #4 {
            n96 = Wait (ms)(milliseconds to wait=w527) -> ()  [unwired: 1 out]
          }
        }
        n97 = case shown="False" w419 {
          selector: w419 -> [_ w500]
          tunnel: [w499 w500] -> w415
          frame False {
            n98 = Two Button Dialog(message="The magnet current is more\nthan 0.1A different to the\nPSU output current.  It is not\nadvisable to switch on the\nswitch heater unless these\ncurrents are equal!") -> (T button?=w499:bool)  [unwired: 2 out]
          }
          frame True {
          }
        }
        n99 = case shown="True" w415 {
          tunnel: w418 -> [w439 w456]
          tunnel: w417 -> [w438 w455]
          tunnel: [w439 w454] -> w413
          tunnel: [w438 w453] -> w412
          tunnel: w416 -> [_ w452]
          tunnel: w414 -> [_ w441]
          tunnel: w414 -> [_ w440]
          frame False {
          }
          frame True {
            n100 = flat-sequence {
              tunnel: [w466] -> w462
              tunnel: [w465] -> w461
              tunnel: [w464] -> w460
              tunnel: w456 -> [w468]
              tunnel: w455 -> [w467]
              tunnel: w452 -> [w463]
              tunnel: [w463] -> w450
              tunnel: w462 -> [w472]
              tunnel: w461 -> [w471]
              tunnel: [w472] -> w459
              tunnel: [w471] -> w458
              tunnel: [w470] -> w457
              tunnel: w460 -> [w470]
              tunnel: [w469] -> w451
              tunnel: w450 -> [w469]
              tunnel: w459 -> [w483]
              tunnel: w458 -> [w484]
              tunnel: w457 -> [w481]
              tunnel: [w478] -> w447
              tunnel: [w479] -> w445
              tunnel: w451 -> [w474]
              tunnel: [w474] -> w443
              tunnel: w447 -> [w488]
              tunnel: [w488] -> w446
              tunnel: w445 -> [w487]
              tunnel: [w487] -> w444
              tunnel: w443 -> [w486]
              tunnel: [w486] -> w442
              tunnel: w441 -> [w485]
              tunnel: w446 -> [w494]
              tunnel: w444 -> [w493]
              tunnel: w442 -> [w489]
              tunnel: [w492] -> w449
              tunnel: [w491] -> w448
              tunnel: [w496] -> w453
              tunnel: [w497] -> w454
              tunnel: w449 -> [w497]
              tunnel: w448 -> [w496]
              tunnel: w440 -> [w495]
              frame #0 {
                n101 = call-poly "Signals (Read).vi"("ISOBUS address"=w463, "error in"=w467, "Mercury Reference In"=w468) -> ("error out"=w466:errorcluster, "Switch Heater Status"=w464:string, "Mercury Reference Out"=w465:T2)  [unwired: 6 out]
              }
              frame #1 {
                n102 = Wait Until Next ms Multiple(millisecond multiple=u32 100) -> ()  [unwired: 1 out]
              }
              frame #2 {
                n103 = Equal?(x=w481, y="ON") -> (x = y?=w480:bool)
                n104 = Select(t=T12 "OFF" ("Set Switch Heater"), s=w480, f=T12 "ON" ("Set Switch Heater")) -> (s? t:f=w475:T12)
                n105 = call-poly "Signals (Set).vi"("ISOBUS address"=w474, "error in"=w483, "Set Switch Heater"=w475, "Mercury Reference In"=w484) -> ("error out"=w479:errorcluster, "Mercury Reference Out"=w478:T2)  [unwired: 6 out]
              }
              frame #3 {
                n106 = Wait (ms)(milliseconds to wait=w485) -> ()  [unwired: 1 out]
              }
              frame #4 {
                n107 = call-poly "Configuration (Read).vi"("ISOBUS address"=w489, "error in"=w493, "Mercury Reference In"=w494) -> ("error out"=w491:errorcluster, "time stamp"=→"Switch TS":timestamp, "Mercury Reference Out"=w492:T2)  [unwired: 6 out]
              }
              frame #5 {
                n108 = Wait (ms)(milliseconds to wait=w495) -> ()  [unwired: 1 out]
              }
            }
          }
        }
      }
      frame "Set Points" {
        n109 = case shown="True" w539 {
          tunnel: w547 -> [w576 w635]
          tunnel: w546 -> [w575 w634]
          tunnel: [w563 w619] -> w535
          tunnel: [w562 w618] -> w534
          tunnel: w544 -> [w552 _]
          tunnel: w545 -> [w553 _]
          tunnel: w543 -> [_ w604]
          tunnel: w542 -> [_ w605]
          tunnel: w541 -> [w564 w633]
          tunnel: w540 -> [w555 w610]
          tunnel: w538 -> [w549 w607]
          tunnel: w537 -> [w551 w606]
          tunnel: [w548 w603] -> w536
          frame False {
            n110 = Divide(x=w553, y=w551) -> (x/y=w554:dbl)
            n111 = Divide(x=w552, y=w551) -> (x/y=w550:dbl)
            n112 = Bundle By Name(cluster=w549, "Target Field (T)"=w554, "Target Rate (T/min)"=w550) -> (w548:T9)
            n113 = flat-sequence {
              tunnel: w553 -> [w579]
              tunnel: w575 -> [w580]
              tunnel: w576 -> [w581]
              tunnel: [w581] -> w574
              tunnel: [w580] -> w573
              tunnel: [w579] -> w572
              tunnel: [w578] -> w565
              tunnel: w564 -> [w578]
              tunnel: [w577] -> w556
              tunnel: w555 -> [w577]
              tunnel: w574 -> [w588]
              tunnel: w573 -> [w587]
              tunnel: w572 -> [w584]
              tunnel: [w586] -> w571
              tunnel: [w585] -> w570
              tunnel: [w583] -> w566
              tunnel: w565 -> [w583]
              tunnel: [w582] -> w557
              tunnel: w556 -> [w582]
              tunnel: w571 -> [w592]
              tunnel: w570 -> [w591]
              tunnel: [w592] -> w569
              tunnel: [w591] -> w568
              tunnel: [w590] -> w567
              tunnel: w566 -> [w590]
              tunnel: [w589] -> w558
              tunnel: w557 -> [w589]
              tunnel: w569 -> [w599]
              tunnel: w568 -> [w598]
              tunnel: w552 -> [w597]
              tunnel: w567 -> [w594]
              tunnel: [w596] -> w561
              tunnel: [w595] -> w560
              tunnel: [w593] -> w559
              tunnel: w558 -> [w593]
              tunnel: [w601] -> w562
              tunnel: [w602] -> w563
              tunnel: w561 -> [w602]
              tunnel: w560 -> [w601]
              tunnel: w559 -> [w600]
              frame #0 {
                n114 = Wait (ms)(milliseconds to wait=w577) -> ()  [unwired: 1 out]
              }
              frame #1 {
                n115 = call-poly "Signals (Set).vi"("ISOBUS address"=w583, "error in"=w587, "Target Current"=w584, "Mercury Reference In"=w588) -> ("error out"=w585:errorcluster, "Mercury Reference Out"=w586:T2)  [unwired: 1 in, 5 out]
              }
              frame #2 {
                n116 = Wait (ms)(milliseconds to wait=w589) -> ()  [unwired: 1 out]
              }
              frame #3 {
                n117 = call-poly "Signals (Set).vi"("ISOBUS address"=w594, "error in"=w598, "Target Current Rate"=w597, "Mercury Reference In"=w599) -> ("error out"=w595:errorcluster, "Mercury Reference Out"=w596:T2)  [unwired: 1 in, 5 out]
              }
              frame #4 {
                n118 = Wait (ms)(milliseconds to wait=w600) -> ()  [unwired: 1 out]
              }
            }
          }
          frame True {
            n119 = Multiply(x=w605, y=w606) -> (x*y=w609:dbl)
            n120 = Multiply(x=w604, y=w606) -> (x*y=w608:dbl)
            n121 = flat-sequence {
              tunnel: w604 -> [w637]
              tunnel: w633 -> [w638]
              tunnel: w605 -> [w639]
              tunnel: w634 -> [w640]
              tunnel: w635 -> [w641]
              tunnel: [w641] -> w632
              tunnel: [w640] -> w631
              tunnel: [w639] -> w630
              tunnel: [w638] -> w629
              tunnel: [w637] -> w628
              tunnel: [w636] -> w611
              tunnel: w610 -> [w636]
              tunnel: w632 -> [w649]
              tunnel: w631 -> [w648]
              tunnel: w630 -> [w645]
              tunnel: w629 -> [w644]
              tunnel: w628 -> [w643]
              tunnel: [w647] -> w627
              tunnel: [w646] -> w626
              tunnel: [w644] -> w625
              tunnel: [w643] -> w624
              tunnel: [w642] -> w612
              tunnel: w611 -> [w642]
              tunnel: w627 -> [w654]
              tunnel: w626 -> [w653]
              tunnel: w625 -> [w652]
              tunnel: w624 -> [w651]
              tunnel: [w654] -> w623
              tunnel: [w653] -> w622
              tunnel: [w652] -> w621
              tunnel: [w651] -> w620
              tunnel: [w650] -> w613
              tunnel: w612 -> [w650]
              tunnel: w623 -> [w661]
              tunnel: w622 -> [w660]
              tunnel: w621 -> [w658]
              tunnel: w620 -> [w659]
              tunnel: [w658] -> w617
              tunnel: [w657] -> w616
              tunnel: [w656] -> w615
              tunnel: [w655] -> w614
              tunnel: w613 -> [w655]
              tunnel: [w663] -> w619
              tunnel: [w664] -> w618
              tunnel: [w665] -> _
              tunnel: w617 -> [w665]
              tunnel: w616 -> [w664]
              tunnel: w615 -> [w663]
              tunnel: w614 -> [w662]
              frame #0 {
                n122 = Wait (ms)(milliseconds to wait=w636) -> ()  [unwired: 1 out]
              }
              frame #1 {
                n123 = call-poly "Signals (Set).vi"("ISOBUS address"=w644, "error in"=w648, "Target Field"=w645, "Mercury Reference In"=w649) -> ("error out"=w646:errorcluster, "Mercury Reference Out"=w647:T2)  [unwired: 1 in, 5 out]
              }
              frame #2 {
                n124 = Wait (ms)(milliseconds to wait=w650) -> ()  [unwired: 1 out]
              }
              frame #3 {
                n125 = call-poly "Signals (Set).vi"("ISOBUS address"=w658, "error in"=w660, "Target Field Rate"=w659, "Mercury Reference In"=w661) -> ("error out"=w657:errorcluster, "Mercury Reference Out"=w656:T2)  [unwired: 1 in, 5 out]
              }
              frame #4 {
                n126 = Wait (ms)(milliseconds to wait=w662) -> ()  [unwired: 1 out]
              }
            }
            n127 = Bundle By Name(cluster=w607, "Target Current (A)"=w609, "Target Rate (A/min)"=w608) -> (w603:T9)
          }
        }
        n128 = local write "Ramp Controls"(w536) -> ()
      }
    }
    "Status" <- w35
    n129 = Wait Until Next ms Multiple(millisecond multiple=u32 1000) -> ()  [unwired: 1 out]
  }
  "error out" <- w1
